vi "Multiples of 3 or 5 Custom Test.vi"(3 "Error In":errorcluster, 4 "Solution VI":path, 5 "User VI":path) -> (0 "Error Out":errorcluster, 2 "Results":T1={"Id"="", "Score"={"Status"=enum."Passed", "cpu_time"=-1, "max_memory"=-1, "style_score"=-1, "score0"="", "score1"="", "score2"="", "score3"="", "score4"="", "score5"=""}})   [LabVIEW 2013]
uses:
  <vilib>/LabVIEW Hacker/VIChallenge/Private/Grader/Type Defs/Grader Result.ctl
  <vilib>/LabVIEW Hacker/VIChallenge/Private/Type Defs/Database/Score.ctl
  <vilib>/LabVIEW Hacker/VIChallenge/Private/Grader/Type Defs/UTF Status.ctl
  <vilib>/LabVIEW Hacker/VIChallenge/VIChallenge.lvlib
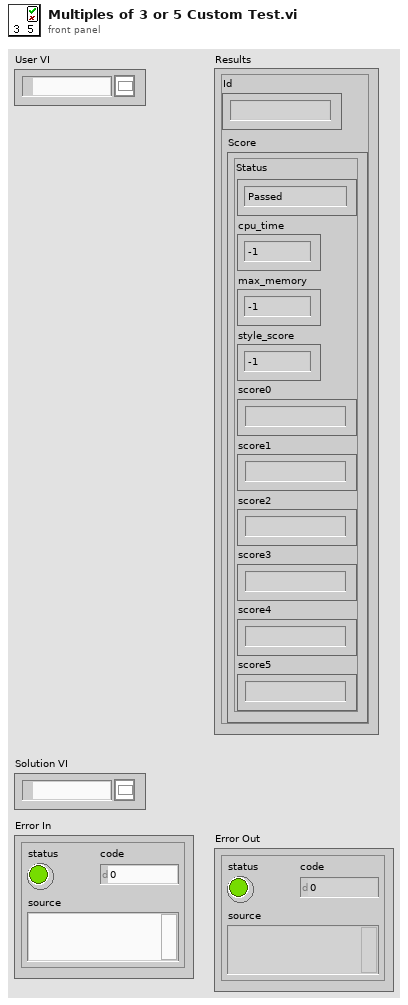
[diagram p1: front panel]
types:
  T1 = typedef "VIChallenge.lvlib/Grader Result.ctl" = cluster{"Id":string, "Score":T2}
  T2 = typedef "VIChallenge.lvlib/Score.ctl" = cluster{"Status":T3, "cpu_time":i32, "max_memory":i32, "style_score":i32, "score0":string, "score1":string, "score2":string, "score3":string, "score4":string, "score5":string}
  T3 = typedef "VIChallenge.lvlib/UTF Status.ctl" = enum16{"Null", "Passed", "Failed", "Error", "Skipped", "Not Processed"}
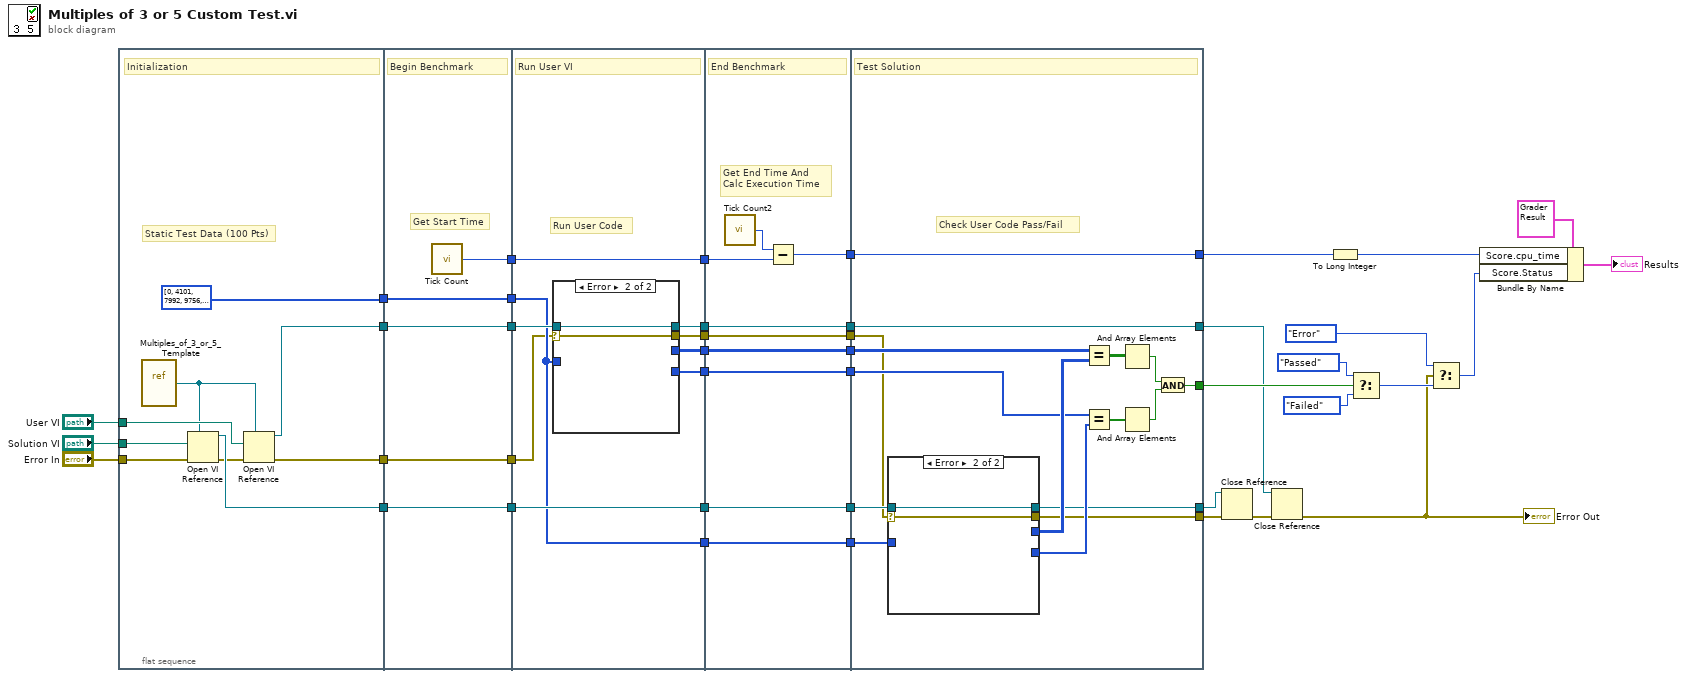
[diagram p0: block diagram]
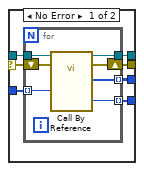
[diagram p2: hidden frame]
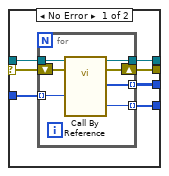
[diagram p3: hidden frame]
diagram:
  n1 = flat-sequence {
    tunnel: [i32[] [0, 4101, 7992, 9756, 2304, 1434, 2642, 763, 8800, 5376, 4574, 363, 6871, 189, 4582, 3087, 9835, 6344, 452, 4823, 2650, 7313, 3598, 6148, 693, 7355, 6605, 7449, 5511, 2696, 8847, 2782, 9773, 581, 4356, 2442, 5108, 3659, 7564, 6573, 6570, 9274, 521, 7327, 3459, 45, 1098, 5744, 2868, 6218, 2280, 6064, 1039, 7872, 1724, 1308, 1491, 5729, 1379, 8154, 9406, 5618, 1813, 2549, 1300, 6245, 9733, 9529, 5903, 4926, 3855, 9688, 2768, 5822, 3318, 8023, 5564, 2468, 1887, 3078, 5488, 8171, 3439, 1744, 207, 7138, 8147, 7578, 4530, 5014, 2956, 2648, 854, 8218, 5855, 6698, 70, 5695, 1998, 2553, 9259, 3723, 9906, 3465, 7061, 5112, 1291, 7516, 1553, 1161, 6832, 9208, 1341, 4707, 5029, 5758, 894, 6882, 9613, 6151, 3174, 4849, 9186, 2514, 890, 5565, 5954, 5833, 2349, 1687, 9382, 715, 9437, 3011, 8559, 4286, 150, 1812, 2347, 6453, 1015, 2531, 9463, 1652, 5832, 9366, 5845, 3541, 8488, 3448, 6300, 2250, 1083, 4910, 5332, 1984, 189, 2816, 9981, 7136, 3692, 7235, 8597, 2210, 5243, 4993, 3136, 2482, 7440, 6978, 5915, 8519, 6995, 8037, 7644, 4774, 4260, 3295, 4653, 3737, 9478, 9248, 2289, 176, 701, 5570, 9769, 6747, 2630, 9538, 584, 8415, 9986, 2466, 3176, 5967, 5477, 8901, 1309, 9998, 1045, 7061, 6538, 1900, 3148, 2900, 6887, 4441, 2589, 7792, 6497, 2217, 7468, 3877, 4629, 878, 5699, 4754, 7315, 6834, 7404, 9237, 270, 8140, 8762, 320, 2858, 171, 7468, 8670, 7779, 731, 8845, 9638, 405, 9333, 555, 3807, 5860, 8289, 4455, 4675, 8465, 2451, 1647, 1590, 9077, 872, 3995, 9718, 1414, 2919, 152, 2947, 609, 7831, 4488, 5089, 214, 9663, 4888, 5656, 4206, 9721, 1241, 4285, 5677, 9831, 615, 5357, 9516, 3879, 1823, 904, 7669, 8173, 2801, 6101, 3841, 5418, 6240, 1509, 5257, 6690, 7816, 9422, 1305, 2228, 7611, 999, 8397, 4302, 257, 3905, 7736, 8495, 294, 5689, 80, 1809, 451, 2319, 6033, 9873, 5398, 2986, 3722, 3972, 3375, 3482, 1767, 2095, 1140, 2097, 4475, 2434, 5460, 3803, 2260, 2882, 5042, 4640, 2436, 2921, 415, 9312, 7868, 2646, 4149, 5293, 8351, 7121, 1624, 9262, 8072, 6069, 5161, 7303, 2181, 4762, 5821, 4336, 8144, 1826, 3607, 9761, 9028, 6103, 9990, 1112, 9431, 8541, 9351, 766, 3179, 300, 663, 9248, 4926, 8967, 5786, 1346, 36, 7738, 2376, 2667, 5098, 5940, 3435, 5423, 4963, 6628, 108, 6928, 8233, 2316, 9614, 2649, 8754, 5432, 3542, 2351, 7233, 8895, 6929, 2421, 5728, 9208, 3437, 7536, 3449, 2124, 1581, 5442, 996, 5109, 5105, 3245, 6449, 9251, 140, 6852, 5064, 892, 5668, 4031, 7352, 4747, 5510, 5376, 4916, 8075, 9013, 7762, 5244, 4385, 926, 5744, 1293, 7678, 5817, 9240, 3243, 6070, 1026, 7547, 9337, 8650, 6167, 5232, 3411, 3637, 8498, 2738, 2931, 2890, 4870, 7482, 2166, 4460, 9204, 606, 1243, 7236, 2325, 7336, 6890, 513, 5885, 5491, 4040, 1014, 5133, 355, 983, 8780, 195, 5711, 4867, 7712, 9553, 428, 8828, 8578, 2014, 7345, 7268, 1259, 6574, 5916, 6866, 8898, 635, 7064, 5190, 5101, 5372, 5960, 1037, 1132, 4149, 6892, 5602, 8354, 6073, 8819, 3580, 3164, 7387, 4210, 4106, 5046, 9394, 5161, 9854, 1203, 1687, 2036, 610, 9387, 294, 710, 9644, 6088, 11, 1417, 9088, 7363, 6956, 6333, 375, 2439, 331, 3595, 599, 4634, 4040, 7736, 2933, 3008, 8351, 5957, 369, 8284, 9933, 1302, 4731, 1251, 1246, 9477, 1242, 4241, 8219, 5884, 3033, 7958, 363, 2913, 9257, 5939, 5596, 2991, 1679, 6995, 7371, 7963, 533, 5709, 4971, 8276, 7692, 4993, 1863, 7300, 8069, 6361, 8833, 6420, 2705, 2946, 533, 2447, 7493, 2870, 8159, 9863, 4594, 93, 4667, 8200, 6926, 3835, 2027, 8399, 7112, 9530, 1933, 1109, 1394, 6647, 4140, 4299, 8964, 4962, 4818, 6398, 7900, 3471, 6760, 2483, 2830, 8359, 6587, 4399, 4853, 2226, 492, 8639, 2372, 4487, 6463, 9958, 7316, 4783, 2888, 9098, 8927, 6773, 5265, 7511, 2768, 8757, 975, 427, 8255, 9665, 5852, 9092, 3889, 6539, 1578, 561, 617, 271, 716, 855, 6807, 5448, 9240, 7264, 6701, 4081, 4590, 2384, 5376, 3557, 8687, 5815, 8348, 4110, 4880, 4812, 7743, 7250, 2469, 3640, 4075, 5515, 1897, 5589, 3889, 5236, 6792, 4111, 2458, 4239, 9765, 7378, 8463, 6523, 412, 8840, 6522, 5305, 7599, 8099, 2982, 5183, 1480, 6570, 4510, 1066, 7407, 2959, 2581, 175, 4666, 3419, 7019, 9152, 3711, 6539, 9138, 3188, 6625, 7568, 1674, 9713, 3107, 7554, 923, 487, 2049, 7303, 4673, 1382, 4900, 3277, 797, 8380, 4567, 9399, 4901, 7196, 4387, 6919, 6428, 4239, 3737, 1167, 6944, 7322, 3611, 5017, 6383, 4829, 2561, 367, 1463, 8986, 6146, 9960, 7919, 3916, 6183, 1797, 9263, 402, 9081, 4001, 3013, 9009, 3702, 3237, 2770, 506, 3880, 8663, 3791, 1003, 800, 4253, 1828, 8875, 7763, 7064, 455, 2634, 8455, 4315, 8212, 4243, 7922, 9287, 6445, 493, 4898, 3078, 7555, 597, 8724, 3871, 864, 5443, 1154, 8333, 7331, 3245, 8179, 21, 6111, 753, 8293, 5369, 1776, 1620, 9990, 8165, 8006, 7343, 5765, 5018, 4698, 4678, 5154, 6095, 8578, 8399, 3154, 2546, 8907, 2585, 9497, 8085, 6184, 9240, 2470, 342, 2849, 9699, 2088, 4626, 8093, 9031, 469, 8144, 2916, 2561, 972, 172, 9762, 2316, 6577, 234, 2053, 4217, 2095, 5197, 982, 4884, 2927, 6918, 2579, 3170, 1276, 8952, 8792, 2759, 7261, 6469, 3139, 8925, 7019, 5950, 6536, 9380, 1189, 7815, 42, 7567, 7641, 9605, 2925, 8338, 7129, 9719, 3011, 1496, 6265, 3069, 6931, 1984, 4492, 4289, 497, 1449, 820, 8883, 3464, 8987, 2028, 9519, 3714, 8020, 3473, 3105, 5875, 1159, 9726, 2470, 430, 9440, 7529, 1225, 5233, 2741, 4649, 8477, 7288, 7380, 3300, 8452, 9972, 3520, 8917, 633, 9234, 3439, 9547, 6489, 5868, 3488, 6977, 8578, 9094, 2436, 1390, 2324, 9486, 7443, 6857, 6310, 1979, 4067, 5560, 2497, 3451, 8093, 9, 9728, 5928, 1317, 8416, 4888, 8557, 2532, 3831, 5252, 6861, 6323, 7914, 8615, 7112, 5793, 4143, 3976, 7217, 8104, 173, 5240, 9005, 8425, 9292, 2707, 264, 672, 4277, 7663, 5538, 5254, 1017, 7713, 8558, 5001, 5345, 4181, 9274, 9471, 56, 8767, 3781, 994, 65, 3872, 6653, 1242, 7179, 8046, 4543, 5442, 7661, 6259, 6321, 2762, 8278, 4784, 8027, 5141, 5654, 3834, 8751, 6653, 4614, 6283, 6354, 9468, 2548, 1877, 9703, 4216, 156, 4113, 3576, 1735, 114, 57, 1289, 6342, 9391, 5588, 2087, 1522, 8049, 6836, 613, 3715, 4907, 7605, 6226, 6503] ("Array")] -> w40
    tunnel: "User VI" -> [w50]
    tunnel: [w49] -> w38
    tunnel: "Solution VI" -> [w48]
    tunnel: [w47] -> w27
    tunnel: "Error In" -> [w45]
    tunnel: [w43] -> w16
    tunnel: [w55] -> w41
    tunnel: w40 -> [w55]
    tunnel: w38 -> [w54]
    tunnel: [w54] -> w37
    tunnel: [w53] -> w32
    tunnel: [w52] -> w28
    tunnel: w27 -> [w52]
    tunnel: w16 -> [w51]
    tunnel: [w51] -> w15
    tunnel: w41 -> [w59]
    tunnel: w37 -> [w64]
    tunnel: [w63] -> w36
    tunnel: [w62] -> w35
    tunnel: [w61] -> w33
    tunnel: w32 -> [w61]
    tunnel: [w60] -> w29
    tunnel: w28 -> [w60]
    tunnel: [w59] -> w26
    tunnel: w15 -> [w56]
    tunnel: [w58] -> w13
    tunnel: [w57] -> w7
    tunnel: w36 -> [w85]
    tunnel: w35 -> [w84]
    tunnel: w33 -> [w89]
    tunnel: [w88] -> w31
    tunnel: [w87] -> w30
    tunnel: w29 -> [w87]
    tunnel: w26 -> [w86]
    tunnel: [w86] -> w25
    tunnel: [w85] -> w24
    tunnel: [w84] -> w23
    tunnel: [w82] -> w14
    tunnel: w13 -> [w82]
    tunnel: [w81] -> w8
    tunnel: w7 -> [w81]
    tunnel: w31 -> [w105]
    tunnel: [w105] -> w5
    tunnel: w30 -> [w104]
    tunnel: w25 -> [w103]
    tunnel: w24 -> [w102]
    tunnel: w23 -> [w99]
    tunnel: [w93] -> w21
    tunnel: w14 -> [w90]
    tunnel: [w96] -> w12
    tunnel: [w95] -> w10
    tunnel: [w94] -> w9
    tunnel: w8 -> [w94]
    frame #0 {
      # "Static Test Data (100 Pts)"
      # "Initialization"
      n2 = vi-ref <vilib>:"Multiples_of_3_or_5_Template.vi"() -> (w46:refnum<vi>)
      n3 = Open VI Reference(type specifier VI Refnum (for type only)=w46, vi path=w48, error in (no error)=w45) -> (vi reference=w47:refnum<vi>, error out=w44:errorcluster)  [unwired: 3 in]
      n4 = Open VI Reference(type specifier VI Refnum (for type only)=w46, vi path=w50, error in (no error)=w44) -> (vi reference=w49:refnum<vi>, error out=w43:errorcluster)  [unwired: 3 in]
    }
    frame #1 {
      # "Get Start Time"
      # "Begin Benchmark"
      n5 = call "Tick Count"() -> ("Tick Count(uSec)"=w53:u32)
    }
    frame #2 {
      # "Run User Code"
      # "Run User VI"
      n6 = case shown="Error" w56 {
        selector: w56 -> [w65 w80]
        tunnel: w64 -> [w71 w79]
        tunnel: [w70 _] -> w63
        tunnel: [w69 _] -> w62
        tunnel: w59 -> [w68 _]
        tunnel: [w67 w80] -> w58
        tunnel: [w66 w79] -> w57
        frame No Error {
          n7 = for {
            tunnel: w71 -> [w78]
            tunnel: w68 -> [w77] mode=indexing
            tunnel: [w76] -> w70 mode=indexing
            tunnel: [w75] -> w69 mode=indexing
            shift-right: [w73] -> w67
            shift-left: w65 -> [w74]
            tunnel: [w72] -> w66
            n8 = call-by-ref "?"(reference=w78, error in=w74, "Maximum"=w77) -> (reference out=w72:refnum<vi>, error out=w73:errorcluster, "Sum"=w75:i32, "Multiples"=w76:i32[])  [unwired: 3 in]
          }
        }
        frame Error {
        }
      }
    }
    frame #3 {
      # "Get End Time And \nCalc Execution Time"
      # "End Benchmark"
      n9 = call "Tick Count2"() -> ("Tick Count(uSec)"=w83:u32)
      n10 = Subtract(x=w83, y=w89) -> (x-y=w88:u32)
    }
    frame #4 {
      # "Check User Code Pass/Fail"
      # "Test Solution"
      n11 = case shown="Error" w90 {
        selector: w90 -> [w106 w121]
        tunnel: w104 -> [w112 w120]
        tunnel: w103 -> [w111 _]
        tunnel: [w110 _] -> w101
        tunnel: [w109 _] -> w100
        tunnel: [w108 w121] -> w96
        tunnel: [w107 w120] -> w95
        frame No Error {
          n12 = for {
            tunnel: w112 -> [w119]
            tunnel: w111 -> [w118] mode=indexing
            tunnel: [w117] -> w110 mode=indexing
            tunnel: [w116] -> w109 mode=indexing
            shift-right: [w114] -> w108
            shift-left: w106 -> [w115]
            tunnel: [w113] -> w107
            n13 = call-by-ref "?"(reference=w119, error in=w115, "Maximum"=w118) -> (reference out=w113:refnum<vi>, error out=w114:errorcluster, "Sum"=w116:i32, "Multiples"=w117:i32[])  [unwired: 3 in]
          }
        }
        frame Error {
        }
      }
      n14 = Equal?(x=w102, y=w101) -> (x = y?=w98:bool[][])
      n15 = Equal?(x=w99, y=w100) -> (x = y?=w97:bool[])
      n16 = And Array Elements(Boolean array=w98) -> (logical AND=w92:bool)
      n17 = And Array Elements(Boolean array=w97) -> (logical AND=w91:bool)
      n18 = And(x=w92, y=w91) -> (x .and. y?=w93:bool)
    }
  }
  n19 = Close Reference(reference=w10, error in (no error)=w12) -> (error out=w11:errorcluster)
  n20 = Close Reference(reference=w9, error in (no error)=w11) -> (error out=w3:errorcluster)
  "Error Out" <- w3
  n21 = To Long Integer(number=w5) -> (32bit integer=w6:i32)
  n22 = Select(t=UTF_Status."Passed" ("Score.Status"), s=w21, f=UTF_Status."Failed" ("Score.Status")) -> (s? t:f=w4:T3)
  n23 = Select(t=UTF_Status."Error", s=w3, f=w4) -> (s? t:f=w2:T3)
  n24 = Bundle By Name(cluster=T1 {"Id"="", "Score"={"Status"=enum."Passed", "cpu_time"=-1, "max_memory"=-1, "style_score"=-1, "score0"="", "score1"="", "score2"="", "score3"="", "score4"="", "score5"=""}} ("Grader Result (Error)"), "Score.cpu_time"=w6, "Score.Status"=w2) -> (→"Results":T1)
